vi "Treat Entity Name.vi"(8 "error in":errorcluster, 10 "Data Name":string) -> (0 "error out":errorcluster, 1 "contains raw xml?":bool, 2 "Entity Name":string)   [LabVIEW 2011]
panel:
  # "Copyright © 2006 James Kring, Inc. All rights reserved.\n\nAuthor: Jim Kring <jim.kring@jameskring.com>\n\nThis library is provided \"AS IS\" , WITHOUT WARRANTIES OR \nCONDITIONS OF ANY KIND, either express or implied.\n\nJames Kring, Inc. -- http://www.jameskring.com"
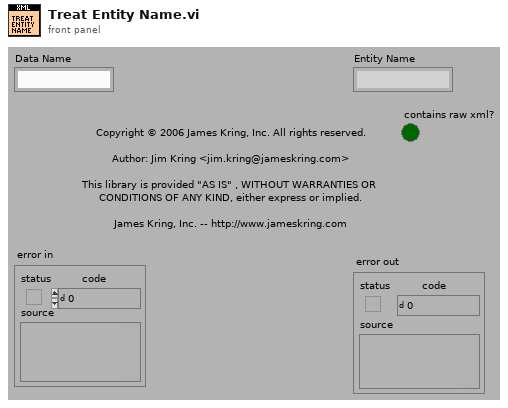
[diagram p1: front panel]
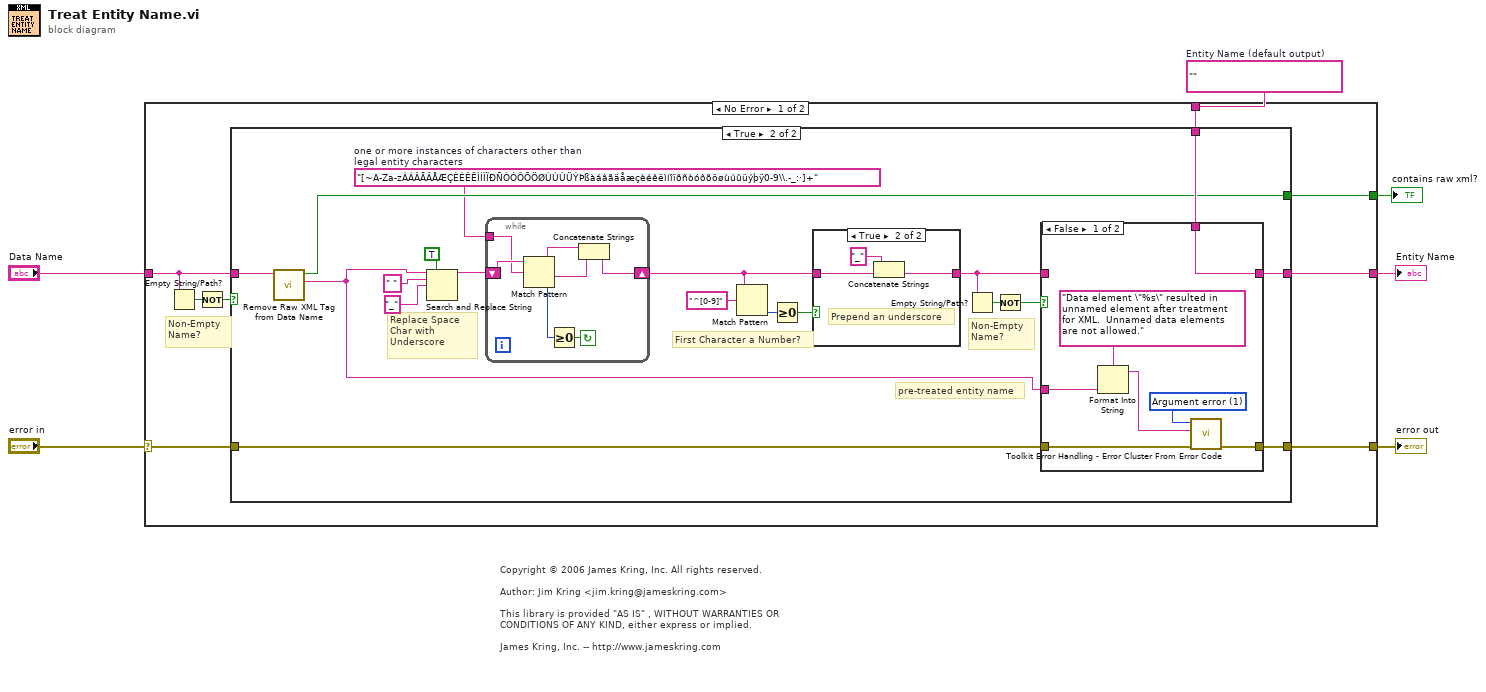
[diagram p0: block diagram]
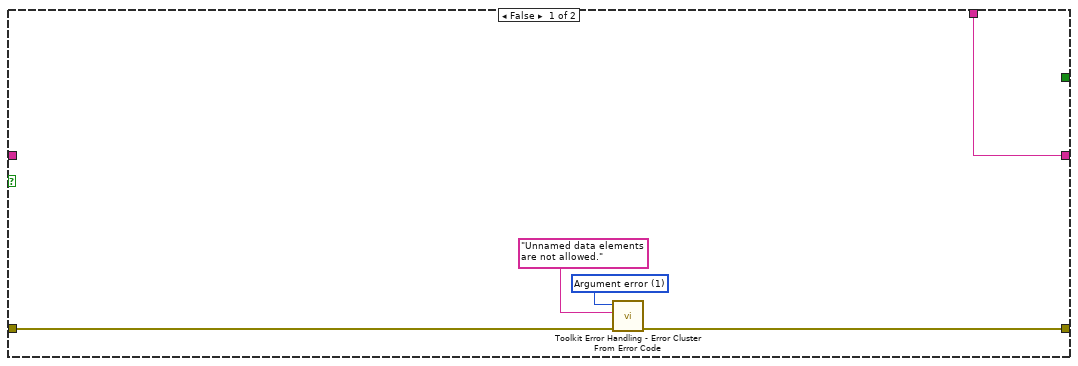
[diagram p2: hidden frame]
diagram:
  w2 = ""  # Entity Name (default output)
  # "Copyright © 2006 James Kring, Inc. All rights reserved.\n\nAuthor: Jim Kring <jim.kring@jameskring.com>\n\nThis library is provided \"AS IS\" , WITHOUT WARRANTIES OR \nCONDITIONS OF ANY KIND, either express or implied.\n\nJames Kring, Inc. -- http://www.jameskring.com"
  n1 = case shown="No Error" "error in" {
    selector: "error in" -> [w10 w59]
    tunnel: [w14 w60] -> w6
    tunnel: [w13 w59] -> w5
    tunnel: "Data Name" -> [w11 _]
    tunnel: w2 -> [w8 w60]
    tunnel: [w7 _] -> w1
    frame No Error {
      # "Non-Empty\nName?"
      n2 = Empty String/Path?(string/path=w11) -> (empty?=w12:bool)
      n3 = Not(x=w12) -> (.not. x?=w9:bool)
      n4 = case shown="True" w9 {
        tunnel: [w15 w26] -> w14
        tunnel: [w16 w29] -> w13
        tunnel: w11 -> [_ w23]
        tunnel: w10 -> [w17 w27]
        tunnel: w8 -> [w15 w25]
        tunnel: [_ w21] -> w7
        frame False {
          w19 = 1 items=["No error", "Argument error", "Memory is full", "Out of zone", "End of file", "File already open", "Generic file I/O error", "File not found", "File permission error", "Disk is full", "Duplicate path", "Too many files open", "System feature not enabled", "Resource file not found", "Cannot add resource", "Resource not found", "Image not found", "Image memory error", "Pen does not exist", "Config type invalid", "Config token not found", "Config parse error", "Config memory error", "Bad external code format", "Bad external code offset", "External code not present", "Null window", "Destroy window error", "Null menu", "Print aborted", "Bad print record", "Print driver error", "Windows error during printing", "Memory error during printing", "Print dialog error", "Generic print error", "Invalid device refnum", "Device not found", "Device parameter error", "Device unit error", "Cannot open device", "Device call aborted", "Generic error", "Cancelled by user", "Object ID too low", "Object ID too high", "Object not in heap", "Unknown heap", "Unknown object (invalid DefProc)", "Unknown object (DefProc not in table)", "Message out of range", "Invalid (null) method", "Unknown message", "Manager call not supported", "Bad address", "Network operation in progress", "Network operation timed out", "Connection is busy", "Network attribute not supported", "Network error", "Address in use", "System out of memory", "Connection aborted", "Connection refused", "Not connected", "Already connected", "Connection closed", "Initialization error (interapplication manager)", "Bad occurrence", "Wait on unbound occurrence handler", "Occurrence queue overflow", "Datalog type conflict", "Unused", "Unrecognized type (interapplication manager)", "Memory corrupt", "Failed to make temporary DLL", "Old CIN version", "Drag socket not found", "Failed to load drop-object", "Failed to register OLE object", "Failed to release OLE object", "Format specifier type mismatch", "Unknown format specifier", "Too few format specifiers", "Too many format specifiers", "Scan failed", "Newer CIN version", "Error converting to variant", "Runtime menu error", "Password tampered", "Variant attribute not found", "Incompatible variant data type", "Event data is not available", "Event Store is not present", "Occurrence is not found", "Event Queue is not created", "Event info is not available", "Refnum passed is NULL", "Error retrieving Class GUID", "Error retrieving CoClass GUID", "Error retrieving TypeLib GUID.", "Bad built application magic bytes.", "Specific driver is different from the specific driver associated with the Logical Name.", "There is no session opened to the class driver.", "Max Error", "MAX - Error with config objects", "MAX - Error loading configuration", "MAX - Group not supported"]
          n5 = call "Toolkit Error Handling - Error Cluster From Error Code.vi"("error in"=w17, "error message (\"\")"="Unnamed data elements are not allowed.", "error code (0)"=w19) -> ("error out"=w16:errorcluster)  [unwired: 6 in]
        }
        frame True {
          w20 = "[~A-Za-zÀÁÂÃÄÅÆÇÈÉÊËÌÍÎÏÐÑÒÓÔÕÖØÙÚÛÜÝÞßàáâãäåæçèéêëìíîïðñòóôõöøùúûüýþÿ0-9\\.-_:·]+"  # one or more instances of characters other than legal entity characters
          # "pre-treated entity name"
          # "Non-Empty\nName?"
          # "Replace Space Char with Underscore"
          # "First Character a Number?"
          n6 = call "Remove Raw XML Tag from Data Name.vi"("Data Name"=w23) -> ("Data Name without #xml"=w22:string, "Raw XML?"=w21:bool)  [unwired: 9 in]
          n7 = Search and Replace String(replace all?=TRUE ("replace all? (F)"), input string=w22, search string=" ", replace string="_" ("replace string (\"\")")) -> (result string=w34:string)  [unwired: 4 in, 3 out]
          n8 = while {
            tunnel: w20 -> [w48]
            shift-right: [w50] -> w35
            shift-left: w34 -> [w49]
            stop <- w54 continue-if-true
            n9 = Match Pattern(string=w49, regular expression=w48) -> (before substring=w52:string, after substring=w51:string, offset past match=w53:i32)  [unwired: 1 in, 1 out]
            n10 = Greater Or Equal To 0?(x=w53) -> (x >= 0?=w54:bool)
            n11 = Concatenate Strings(w52, w51) -> (w50:string)
          }
          n12 = Match Pattern(string=w35, regular expression="^[0-9]") -> (offset past match=w37:i32)  [unwired: 1 in, 3 out]
          n13 = Greater Or Equal To 0?(x=w37) -> (x >= 0?=w36:bool)
          n14 = case shown="True" w36 {
            tunnel: w35 -> [w55 w58]
            tunnel: [w55 w56] -> w24
            frame False {
            }
            frame True {
              # "Prepend an underscore"
              n15 = Concatenate Strings("_" ("string"), w58) -> (w56:string)
            }
          }
          n16 = Empty String/Path?(string/path=w24) -> (empty?=w30:bool)
          n17 = Not(x=w30) -> (.not. x?=w28:bool)
          n18 = case shown="False" w28 {
            tunnel: [w43 w47] -> w29
            tunnel: w27 -> [w44 w47]
            tunnel: [w42 w46] -> w26
            tunnel: w25 -> [w42 _]
            tunnel: w24 -> [_ w46]
            tunnel: w22 -> [w41 _]
            frame False {
              w45 = 1 items=["No error", "Argument error", "Memory is full", "Out of zone", "End of file", "File already open", "Generic file I/O error", "File not found", "File permission error", "Disk is full", "Duplicate path", "Too many files open", "System feature not enabled", "Resource file not found", "Cannot add resource", "Resource not found", "Image not found", "Image memory error", "Pen does not exist", "Config type invalid", "Config token not found", "Config parse error", "Config memory error", "Bad external code format", "Bad external code offset", "External code not present", "Null window", "Destroy window error", "Null menu", "Print aborted", "Bad print record", "Print driver error", "Windows error during printing", "Memory error during printing", "Print dialog error", "Generic print error", "Invalid device refnum", "Device not found", "Device parameter error", "Device unit error", "Cannot open device", "Device call aborted", "Generic error", "Cancelled by user", "Object ID too low", "Object ID too high", "Object not in heap", "Unknown heap", "Unknown object (invalid DefProc)", "Unknown object (DefProc not in table)", "Message out of range", "Invalid (null) method", "Unknown message", "Manager call not supported", "Bad address", "Network operation in progress", "Network operation timed out", "Connection is busy", "Network attribute not supported", "Network error", "Address in use", "System out of memory", "Connection aborted", "Connection refused", "Not connected", "Already connected", "Connection closed", "Initialization error (interapplication manager)", "Bad occurrence", "Wait on unbound occurrence handler", "Occurrence queue overflow", "Datalog type conflict", "Unused", "Unrecognized type (interapplication manager)", "Memory corrupt", "Failed to make temporary DLL", "Old CIN version", "Drag socket not found", "Failed to load drop-object", "Failed to register OLE object", "Failed to release OLE object", "Format specifier type mismatch", "Unknown format specifier", "Too few format specifiers", "Too many format specifiers", "Scan failed", "Newer CIN version", "Error converting to variant", "Runtime menu error", "Password tampered", "Variant attribute not found", "Incompatible variant data type", "Event data is not available", "Event Store is not present", "Occurrence is not found", "Event Queue is not created", "Event info is not available", "Refnum passed is NULL", "Error retrieving Class GUID", "Error retrieving CoClass GUID", "Error retrieving TypeLib GUID.", "Bad built application magic bytes.", "Specific driver is different from the specific driver associated with the Logical Name.", "There is no session opened to the class driver.", "Max Error", "MAX - Error with config objects", "MAX - Error loading configuration", "MAX - Group not supported"]
              n19 = Format Into String(format string="Data element \"%s\" resulted in unnamed element after treatment for XML.  Unnamed data elements are not allowed.", w41) -> (resulting string=w40:string)  [unwired: 2 in, 1 out]
              n20 = call "Toolkit Error Handling - Error Cluster From Error Code.vi"("error in"=w44, "error message (\"\")"=w40, "error code (0)"=w45) -> ("error out"=w43:errorcluster)  [unwired: 6 in]
            }
            frame True {
            }
          }
        }
      }
    }
    frame Error {
    }
  }
  "Entity Name" <- w6
  "error out" <- w5
  "contains raw xml?" <- w1
